vi "Global 2.vi"() -> ()   [LabVIEW 2014]
panel:
  out "Distance inch":dbl
  out "Scale%":dbl format="%#_3g"
  in  "Toggle On for down":bool
  in  "Toggle On for up":bool
  in  "Toggle Down":bool
  in  "Toggle Up":bool
  in  "Toggle Lights":bool
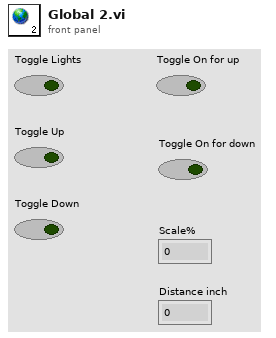
[diagram p1: front panel]
diagram:
